vi "alg_LUDecomposition (SubVI).vi"(0 "A":dbl[][](array[numeric])=[[1.0, 2.0], [3.0, 4.0]], 11 "에러 입력(에러 없음)":errorcluster) -> (4 "참조 번호 출력":refnum<k35>, 6 "L":dbl[][](array[numeric]), 8 "U":dbl[][](array[numeric]), 10 "P":i32[][](array[numeric]), 15 "에러 출력":errorcluster)   [LabVIEW 2018]
uses:
  PythonConfigGlobal.vi
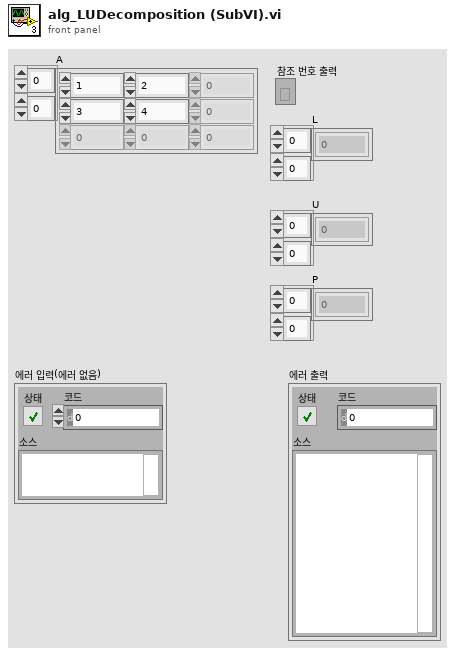
[diagram p1: front panel]
types:
  T1 = cluster{"session out":refnum<k35>, "appended path":path}
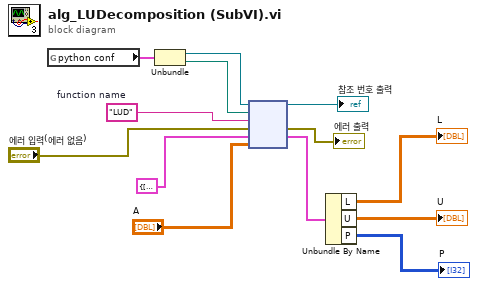
[diagram p0: block diagram]
diagram:
  w2 = "LUD"  # function name
  n1 = global read "PythonConfigGlobal.vi" "python conf"() -> (w5:T1)
  n2 = Unbundle(w5) -> ("session out"=w3:refnum<k35>, "appended path"=w4:path)
  n3 = node(w3, w4, w2, "에러 입력(에러 없음)", cluster{"P":i32[][], "L":dbl[][], "U":dbl[][]} {"P"=[], "L"=[], "U"=[]}, "A") -> (→"참조 번호 출력":refnum<k35>, →"에러 출력":errorcluster, w10:cluster{"P":i32[][], "L":dbl[][], "U":dbl[][]})  [unwired: 1 in, 2 out]
  n4 = Unbundle By Name(w10) -> ("L"=→"L":dbl[][], "U"=→"U":dbl[][], "P"=→"P":i32[][])
